vi "Agilent MXA Series Configure and Query Marker.vi"() -> ()   [LabVIEW 2018]
doc: "This example shows how to configure the spectrum analyzer to query marker."
uses:
  Public/Configure/Configure Frequency (Start Stop).vi
  Public/Configure/Configure Level (Normal).vi
  Public/Configure/Marker/Configure Marker Type (Swept SA).vi
  Agilent MXA Series.lvlib
panel:
  in  "Manual Detector Type (0: Normal)":i32(ring) items=["Normal", "Average", "Peak", "Sample", "Negative peak"]
  out "Marker Amplitude":dbl
  out "Marker Position":dbl
  in  "Marker Search (0: Highest)":i32(ring) items=["Highest", "Next Peak", "Next Peak Left", "Next Peak Right", "Pk-Pk Search", "Minimum"]
  in  "Marker Type (0: Normal)":i32(ring) items=["Normal", "Delta", "Fixed", "Off"]
  in  "Active Marker (1: Marker1)":i32(ring)=1 items=["Marker1"=1, "Marker2"=2, "Marker3"=3, "Marker4"=4, "Marker5"=5, "Marker6"=6, "Marker7"=7, "Marker8"=8, "Marker9"=9, "Marker10"=10, "Marker11"=11, "Marker12"=12]
  in  "Reference Level Offset (0 dB)":dbl
  in  "Reference Level (10 dBm)":dbl=10.0
  in  "Input Impedance (0: 50 ohms)":i32(ring) items=["50", "75"]
  in  "Stop Frequency (25 E+9 Hz)":dbl=25000000000.0
  in  "Start Frequency (100 E+3 Hz)":dbl=100000.0
  in  "VISA resource name":refnum<visa-resource-name>
  # "(c) 2007-2015 National Instruments.  ALL RIGHTS RESERVED."
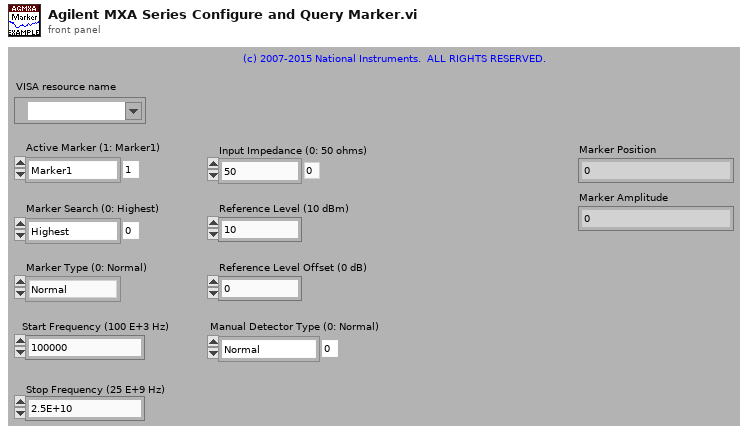
[diagram p1: front panel]
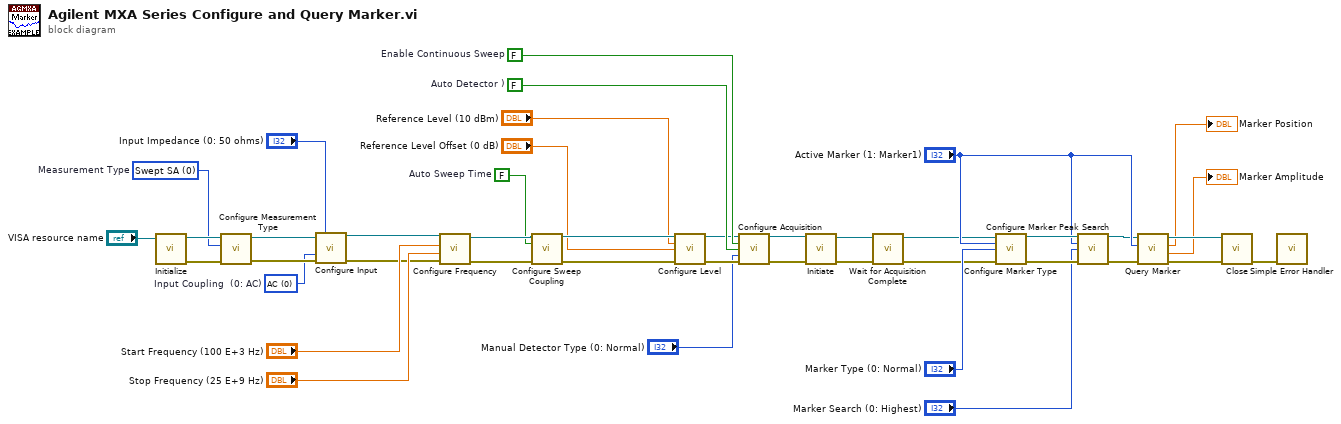
[diagram p0: block diagram]
diagram:
  w28 = 0 items=["AC", "DC"]  # Input Coupling  (0: AC)
  w34 = 0 items=["Swept SA", "Channel Power", "Occupied Bandwidth", "Power Stat CCDF", "Adjacent Channel Power", "Burst Power", "Spurious Emissions", "Spectrum Emission Mask", "List Sweep"]  # Measurement Type
  w33 = FALSE  # Auto Sweep Time
  w32 = FALSE  # Auto Detector )
  w31 = FALSE  # Enable Continuous Sweep
  n1 = call "Initialize.vi"("VISA resource name"="VISA resource name") -> ("error out"=w37:errorcluster, "VISA resource name out"=w38:refnum<visa-resource-name>)  [unwired: 9 in]
  n2 = call "Configure Measurement Type.vi"("error in (no error)"=w37, "Measurement Type (0: Swept SA)"=w34, "VISA resource name"=w38) -> ("error out"=w29:errorcluster, "VISA resource name out"=w30:refnum<visa-resource-name>)  [unwired: 7 in]
  n3 = call "Configure Input.vi"("VISA resource name"=w30, "Input Impedance (0: 50 ohms)"="Input Impedance (0: 50 ohms)", "Input Coupling  (0: AC)"=w28, "error in (no error)"=w29) -> ("VISA resource name out"=w18:refnum<visa-resource-name>, "error out"=w17:errorcluster)  [unwired: 10 in]
  n4 = call-poly "Configure Frequency.vi"("error in (no error)"=w17, "Stop Frequency (2.65E+10 Hz)"="Stop Frequency (25 E+9 Hz)", "Start Frequency (1E+7 Hz)"="Start Frequency (100 E+3 Hz)", "VISA resource name"=w18) -> ("error out"=w35:errorcluster, "VISA resource name out"=w36:refnum<visa-resource-name>)  [unwired: 6 in]
  n5 = call "Configure Sweep Coupling.vi"("VISA resource name"=w36, "Auto Sweep Time (T: Enable)"=w33, "error in (no error)"=w35) -> ("VISA resource name out"=w23:refnum<visa-resource-name>, "error out"=w26:errorcluster)  [unwired: 11 in]
  n6 = call-poly "Configure Level.vi"("VISA resource name"=w23, "Reference Level (0 dBm)"="Reference Level (10 dBm)", "Reference Level Offset (0 dB)"="Reference Level Offset (0 dB)", "error in (no error)"=w26) -> ("VISA resource name out"=w24:refnum<visa-resource-name>, "error out"=w25:errorcluster)  [unwired: 10 in]
  n7 = call "Configure Acquisition.vi"("VISA resource name"=w24, "Enable Continuous Sweep (T: Enable)"=w31, "Auto Detector (T: Enable)"=w32, "Manual Detector Type (0: Normal)"="Manual Detector Type (0: Normal)", "error in (no error)"=w25) -> ("VISA resource name out"=w7:refnum<visa-resource-name>, "error out"=w6:errorcluster)  [unwired: 9 in]
  n8 = call "Initiate.vi"("error in (no error)"=w6, "VISA resource name"=w7) -> ("error out"=w10:errorcluster, "VISA resource name out"=w11:refnum<visa-resource-name>)  [unwired: 8 in]
  n9 = call "Wait for Acquisition Complete.vi"("error in (no error)"=w10, "VISA resource name"=w11) -> ("error out"=w4:errorcluster, "VISA resource name out"=w5:refnum<visa-resource-name>)  [unwired: 8 in]
  n10 = call-poly "Configure Marker Type.vi"("VISA resource name"=w5, "Active Marker (1: Marker1)"="Active Marker (1: Marker1)", "Marker Type (0: Normal)"="Marker Type (0: Normal)", "error in (no error)"=w4) -> ("VISA resource name out"=w20:refnum<visa-resource-name>, "error out"=w19:errorcluster)  [unwired: 10 in]
  n11 = call "Configure Marker Peak Search.vi"("VISA resource name"=w20, "Active Marker (1: Marker1)"="Active Marker (1: Marker1)", "Marker Search (0: Highest)"="Marker Search (0: Highest)", "error in (no error)"=w19) -> ("VISA resource name out"=w9:refnum<visa-resource-name>, "error out"=w8:errorcluster)  [unwired: 10 in]
  n12 = call "Query Marker.vi"("error in (no error)"=w8, "Active Marker (1: Marker1)"="Active Marker (1: Marker1)", "VISA resource name"=w9) -> ("error out"=w21:errorcluster, "Marker Amplitude"=→"Marker Amplitude":dbl, "Marker Position"=→"Marker Position":dbl, "VISA resource name out"=w22:refnum<visa-resource-name>)  [unwired: 5 in]
  n13 = call "Close.vi"("error in (no error)"=w21, "VISA resource name"=w22) -> ("error out"=w42:errorcluster)  [unwired: 9 in]
  n14 = call <vilib>:"Simple Error Handler.vi"("error in (no error)"=w42) -> ()  [unwired: 4 in, 5 out]
